vi "Go to Filter Wheel Start Position.vi"(0 "Session Handle in":T1, 11 "error in (no error)":errorcluster) -> (4 "Session Handle out":T1, 15 "error out":errorcluster)   [LabVIEW 2015, in "PAS.lvclass"]
uses:
  PAS.lvclass
  Typedefs/Session Handle.ctl
panel:
  out "Success?":bool
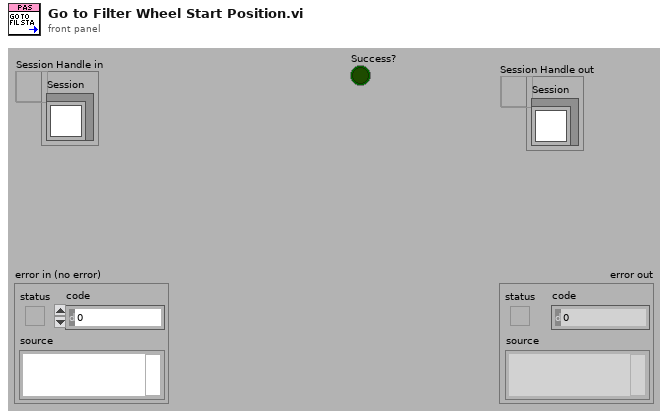
[diagram p1: front panel]
types:
  T1 = typedef "PAS.lvclass/Session Handle.ctl" = refnum<data-value>
  T2 = typedef "XNET Frame CAN.ctl" = cluster{"timestamp":timestamp, "payload":u8[], "identifier":u32, "type":T3, "extended?":bool, "echo?":bool}
  T3 = typedef "XNET Frame Type CAN.ctl" = u8
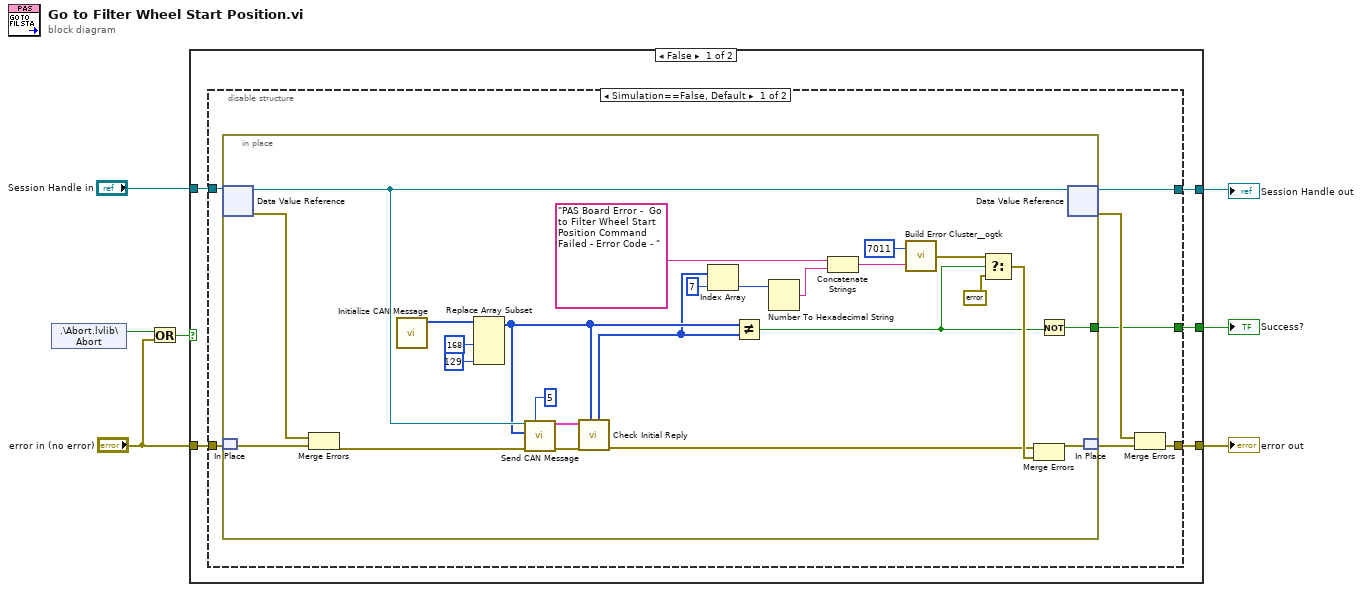
[diagram p0: block diagram]
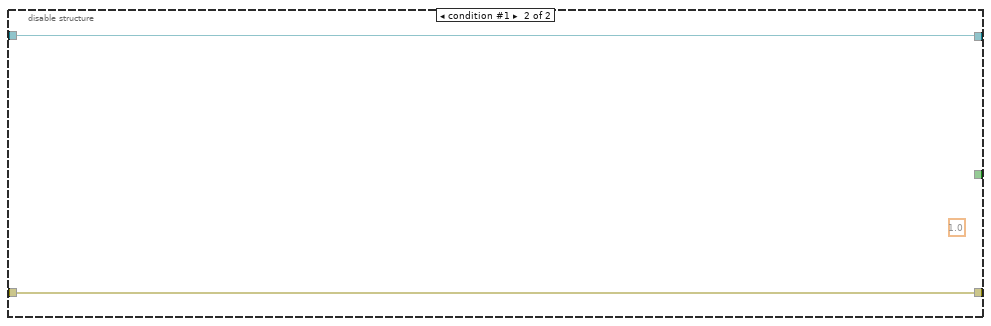
[diagram p2: hidden frame]
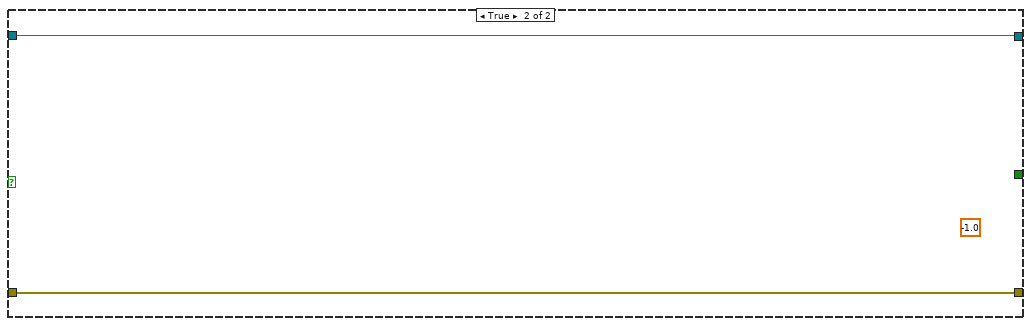
[diagram p3: hidden frame]
diagram:
  n1 = shared-variable ".\\Abort.lvlib\\Abort"() -> (w4:bool)  [unwired: 1 in, 1 out]
  n2 = Or(x=w4, y="error in (no error)") -> (x .or. y?=w2:bool)
  n3 = case shown="False" w2 {
    tunnel: [w12 w48] -> w6
    tunnel: [w11 w47] -> w5
    tunnel: "Session Handle in" -> [w10 w48]
    tunnel: "error in (no error)" -> [w9 w47]
    tunnel: [w8 _] -> w1
    frame False {
      n4 = disable-structure shown="Simulation==False, Default" {
        disable-tunnel: [w19 w46] -> w12
        disable-tunnel: [w16 w45] -> w11
        disable-tunnel: w10 -> [w15 w46]
        disable-tunnel: w9 -> [w14 w45]
        disable-tunnel: [w13 _] -> w8
        frame condition #0 (active) {
          n5 = in-place {
            in-place-border: [w34] -> w13
            n6 = in-place-dvr #1(w15) -> (w37:refnum<class "PAS.lvclass">, w41:errorcluster)
            n7 = in-place-match #2(w14) -> (w40:errorcluster)
            n8 = Merge Errors(w41, w40) -> (w36:errorcluster)
            n9 = call "Initialize CAN Message.vi"() -> ("Initial Payload"=w42:u8[])  [unwired: 11 in]
            n10 = Replace Array Subset(array=w42, new element #1=u8 168 ("new element/subarray"), new element #2=u8 129 ("new element/subarray")) -> (w29:u8[])  [unwired: 2 in]
            n11 = call "Send CAN Message.vi"("Number of Retries"=5, "error in (no error)"=w36, "payload"=w29, "Pas In"=w37) -> ("error out"=w21:errorcluster, "Reply"=w38:T2[])  [unwired: 5 in, 1 out]
            n12 = call "Check Initial Reply.vi"("Write Message"=w29, "error in (no error)"=w21, "Reply"=w38) -> ("error out"=w20:errorcluster, "Whole Payload"=w27:u8[])  [unwired: 5 in, 2 out]
            n13 = Index Array(array=w27, index=7) -> (element=w25:u8)
            n14 = Not Equal?(x=w29, y=w27) -> (x != y?=w28:bool)
            n15 = Number To Hexadecimal String(2:w25) -> (0:w22:string)  [unwired: 1 in]
            n16 = Concatenate Strings("PAS Board Error -  Go to Filter Wheel Start Position Command Failed - Error Code - " ("string"), w22) -> (w23:string)
            n17 = call <userlib>:"Build Error Cluster__ogtk.vi"("String to Prepend to source (\"\")"=w23, "code"=7011) -> ("error out"=w33:errorcluster)
            n18 = Select(t=w33, s=w28, f=errorcluster {"status"=FALSE, "code"=0, "source"=""}) -> (s? t:f=w30:errorcluster)
            n19 = Merge Errors(w20, w30) -> (w43:errorcluster)
            n20 = Not(x=w28) -> (.not. x?=w34:bool)
            n21 = in-place-dvr #1(w37) -> (w19:T1, w17:errorcluster)
            n22 = in-place-match #2(w43) -> (w18:errorcluster)
          }
          n23 = Merge Errors(w17, w18) -> (w16:errorcluster)
        }
        frame condition #1 {
          (unwired) 1.0
        }
      }
    }
    frame True {
      (unwired) -1.0
    }
  }
  "Session Handle out" <- w6
  "error out" <- w5
  "Success?" <- w1
